vi "fpga resource mapping.vi"(8 "error in (no error)":errorcluster, 11 "Node Ptr":T2 format="%.0x") -> (0 "error out":errorcluster)   [LabVIEW 2016, in "FPGA Addon System Explorer.lvlib"]
uses:
  FPGA Addon System Explorer.lvlib
  <vilib>/NI Veristand/Custom Device API/Custom Device Item Ref.ctl
  FPGA-Resource-Manager-APIs/Source/Channel Type.ctl
  <vilib>/NI VeriStand/Custom Device API/Custom Device API.lvlib
  FPGA-Resource-Manager-APIs/Source/System Definition/FPGA RM System Definition API.lvlib
panel:
  out "name pattern":string
  out "datatype":string
  out "channel type":T1
  in  "mapped resource":string(tree)
  in  "Header":cluster{"Section Name":string}={"Section Name"="FPGA Resource Mapping"}
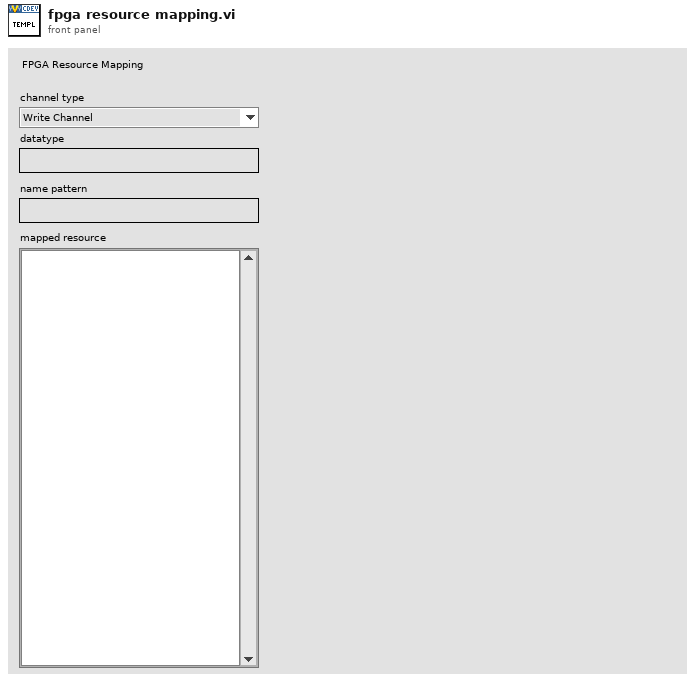
[diagram p1: front panel]
types:
  T1 = typedef "FPGA RM System Definition API.lvlib/Channel Type.ctl" = enum16{"Write Channel", "Read Channel", "Write Waveform", "Read Waveform"}
  T2 = typedef "Custom Device API.lvlib/Custom Device Item Ref.ctl" = u64
  T3 = typedef "Custom Device API.lvlib/Custom Device Commands.ctl" = enum16{"Default", "Item renamed", "Shutdown", "Dynamic button pressed"}
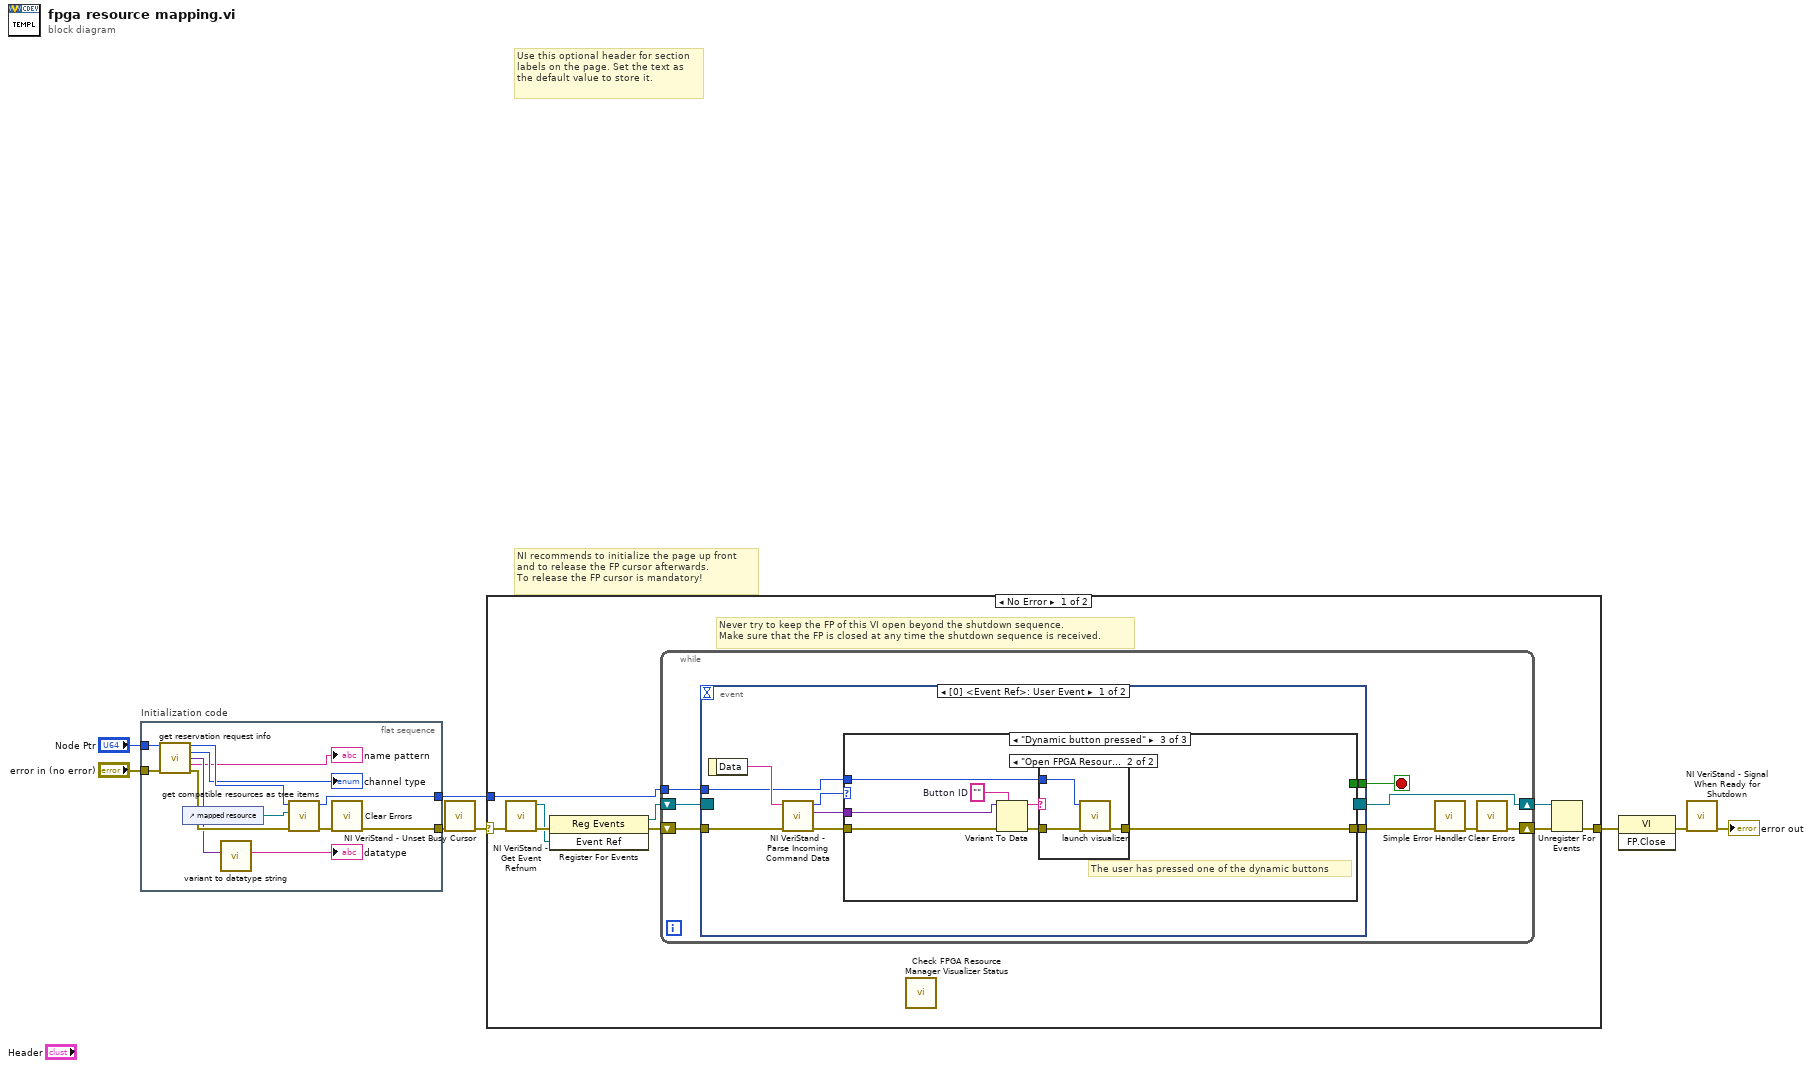
[diagram p0: block diagram]
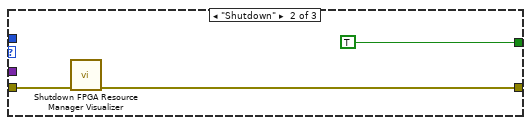
[diagram p3: hidden frame]
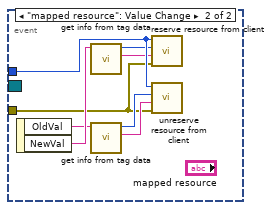
[diagram p5: hidden frame]
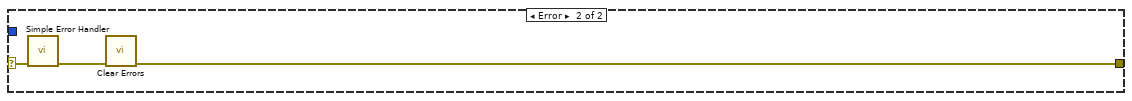
[diagram p6: hidden frame]
diagram:
  # "Use this optional header for section labels on the page. Set the text as the default value to store it."
  # "NI recommends to initialize the page up front\nand to release the FP cursor afterwards.\nTo release the FP cursor is mandatory!"
  n1 = flat-sequence "Initialization code" {
    tunnel: "error in (no error)" -> [w12]
    tunnel: "Node Ptr" -> [w13]
    tunnel: [w20] -> w2
    tunnel: [w11] -> w1
    frame #0 {
      n2 = call "get reservation request info.vi"("Item Ref in"=w13, "error in (no error)"=w12) -> ("Item Ref out"=w17:T2, "channel type"=→"channel type":T1, "datatype"=w16:variant, "Pattern"=→"name pattern":string, "error out"=w18:errorcluster)  [unwired: 9 in]
      n3 = control-ref of="mapped resource"() -> (w10:refnum<vi>)
      n4 = call "variant to datatype string.vi"("Variant"=w16) -> ("datatype string"=→"datatype":string)  [unwired: 9 in, 1 out]
      n5 = call "get compatible resources as tree items.vi"("error in (no error)"=w18, "Tree Refnum"=w10, "Item Ref in"=w17) -> ("error out"=w19:errorcluster, "Item Ref out"=w20:T2)  [unwired: 7 in]
      n6 = call <vilib>:"Clear Errors.vi"("error in (no error)"=w19) -> ("error out"=w11:errorcluster)  [unwired: 5 in, 1 out]
    }
  }
  n7 = call <vilib>:"NI VeriStand - Unset Busy Cursor.vi"("error in (no error)"=w1) -> ("error out"=w4:errorcluster)  [unwired: 10 out]
  n8 = case shown="No Error" w4 {
    selector: w4 -> [w21 w71]
    tunnel: [w26 w69] -> w8
    tunnel: w2 -> [w22 _]
    frame No Error {
      # "Never try to keep the FP of this VI open beyond the shutdown sequence.\nMake sure that the FP is closed at any time the shutdown sequence is received."
      n9 = call <vilib>:"NI VeriStand - Get Event Refnum.vi"("error in (no error)"=w21) -> ("error out"=w29:errorcluster, "Event Ref"=w25:refnum<user-event>)  [unwired: 9 out]
      n10 = register-events(error in=w29, w25) -> (reference out=w23:refnum<event-registration>, error out=w24:errorcluster)  [unwired: 1 in]
      n11 = while {
        tunnel: w22 -> [w33]
        shift-right: [w30] -> w27
        shift-left: w24 -> [w36]
        shift-right: [w37] -> w28
        shift-left: w23 -> [w35]
        stop <- w34 stop-if-true
        n12 = event shown="[0] <Event Ref>: User Event" {
          selector: w35 -> [_ _]
          dyn-events: [_ _] -> w37
          timeout: _ -> [_ _]
          tunnel: w36 -> [w45 w62]
          tunnel: [w41 _] -> w34
          tunnel: [w40 _] -> w32
          tunnel: w33 -> [w39 w68]
          event User Event {
            n13 = event-data() -> ("Data"=w44:string)  [unwired: 1 out]
            n14 = call <vilib>:"NI VeriStand - Parse Incoming Command Data.vi"("error in (no error)"=w45, "Incoming data"=w44) -> ("error out"=w43:errorcluster, "Outgoing data"=w38:variant, "Action"=w42:T3)  [unwired: 7 out]
            n15 = case shown="\"Dynamic button pressed\"" w42 {
              tunnel: w43 -> [w46 w48 w56]
              tunnel: [_ TRUE _] -> w41
              tunnel: [w46 w47 w50] -> w40
              tunnel: w39 -> [_ _ w52]
              tunnel: w38 -> [_ _ w55]
              frame "Default", Default {
              }
              frame "Shutdown" {
                n16 = call "Shutdown FPGA Resource Manager Visualizer.vi"("error in (no error)"=w48) -> ("error out"=w47:errorcluster)  [unwired: 10 in]
              }
              frame "Dynamic button pressed" {
                w54 = ""  # Button ID
                # "The user has pressed one of the dynamic buttons"
                n17 = Variant To Data(error in=w56, type=w54, Variant=w55) -> (data=w53:string, error out=w51:errorcluster)
                n18 = case shown="\"Open FPGA Resource Manager\"" w53 {
                  tunnel: w52 -> [_ w60]
                  tunnel: w51 -> [w57 w59]
                  tunnel: [w57 w58] -> w50
                  frame "False", Default {
                  }
                  frame "Open FPGA Resource Manager" {
                    n19 = call "launch visualizer.vi"("error in (no error)"=w59, "Device Ref in"=w60) -> ("error out"=w58:errorcluster)  [unwired: 8 in, 1 out]
                  }
                }
              }
            }
          }
          event "mapped resource": Value Change {
            n20 = event-data() -> ("OldVal"=w61:string, "NewVal"=w65:string)  [unwired: 1 out]
            n21 = call "get info from tag data.vi"("NewVal"=w65) -> ("item name"=w66:string, "CD ref"=w67:T2)  [unwired: 8 in, 1 out]
            n22 = call "get info from tag data.vi"("NewVal"=w61) -> ("item name"=w63:string, "CD ref"=w64:T2)  [unwired: 8 in, 1 out]
            n23 = call "reserve resource from client.vi"("error in (no error)"=w62, "Name in Bitfile"=w66, "Server Ref in"=w67, "Item Ref in"=w68) -> ()  [unwired: 6 in, 2 out]
            n24 = call "unreserve resource from client.vi"("error in (no error)"=w62, "Name in Bitfile"=w63, "Server Ref in"=w64, "Item Ref in"=w68) -> ()  [unwired: 6 in, 2 out]
          }
        }
        n25 = call <vilib>:"Simple Error Handler.vi"("error in (no error)"=w32) -> ("error out"=w31:errorcluster)  [unwired: 1 in, 7 out]
        n26 = call <vilib>:"Clear Errors.vi"("error in (no error)"=w31) -> ("error out"=w30:errorcluster)  [unwired: 1 in, 5 out]
      }
      n27 = call "Check FPGA Resource Manager Visualizer Status.vi"() -> ()  [unwired: 12 in]
      n28 = Unregister For Events(event registration refnum=w28, error in=w27) -> (error out=w26:errorcluster)
    }
    frame Error {
      n29 = call <vilib>:"Simple Error Handler.vi"("error in (no error)"=w71) -> ("error out"=w70:errorcluster)  [unwired: 1 in, 7 out]
      n30 = call <vilib>:"Clear Errors.vi"("error in (no error)"=w70) -> ("error out"=w69:errorcluster)  [unwired: 1 in, 5 out]
    }
  }
  n31 = invoke class="VI" method="FP.Close"(error in=w8) -> (error out=w7:errorcluster)  [unwired: 2 in, 2 out]
  n32 = call <vilib>:"NI VeriStand - Signal When Ready for Shutdown.vi"("error in (no error)"=w7) -> ("error out"=→"error out":errorcluster)  [unwired: 10 out]
